vi "传感器数据.vi"() -> (0 "电机角度":sgl format="%#.3f", 1 "拉压力":sgl format="%#.3f", 2 "扭矩":sgl format="%#.3f", 3 "电缸位移":sgl format="%#.3f", 4 "电缸自带压力":sgl format="%#.3f", 5 "传感器读数":T1 {"Factorysensor2" format="%#.3f"; "输出轴移栽位移" format="%#.3f"; "输出轴旋转角度" format="%#.3f"; "Factorysensor" format="%#.3f"; "吸收电流" format="%#.3f"; "输出扭矩(大)" format="%#.3f"; "输出扭矩(小)" format="%#.3f"; "扭矩" format="%#.3f"; "输入编码位移" format="%#.3f"; "工装移载位移" format="%#.3f"; "输入移载位移" format="%#.3f"; "输入旋转位移" format="%#.3f"})   [LabVIEW 2020]
uses:
  Libraries/S7/S7.lvlib
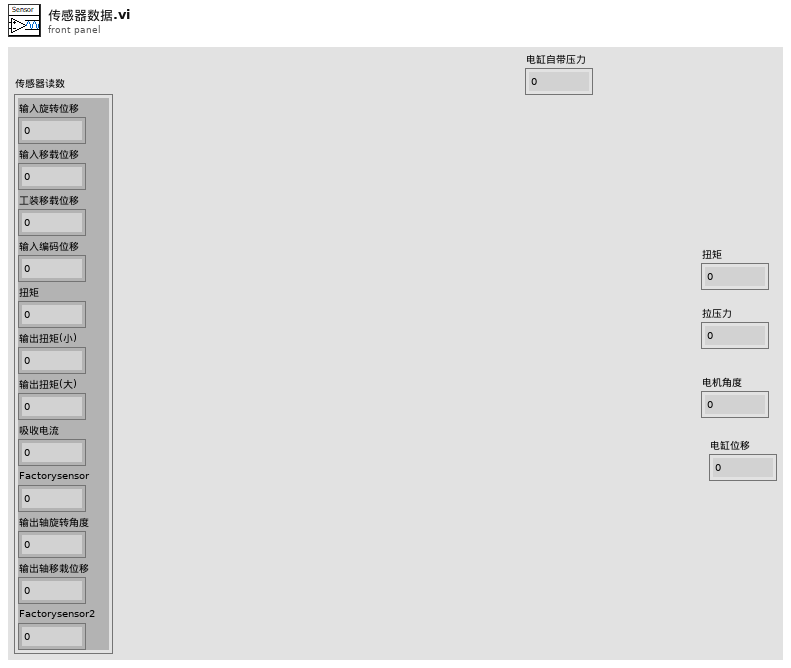
[diagram p1: front panel]
types:
  T1 = cluster{"输入旋转位移":sgl, "输入移载位移":sgl, "工装移载位移":sgl, "输入编码位移":sgl, "扭矩":sgl, "输出扭矩(小)":sgl, "输出扭矩(大)":sgl, "吸收电流":sgl, "Factorysensor":sgl, "输出轴旋转角度":sgl, "输出轴移栽位移":sgl, "Factorysensor2":sgl}
  T2 = cluster{"输入轴扭矩":dbl, "输出轴扭矩小量程":dbl, "输出轴扭矩大量程":dbl}
  T3 = typedef "S7.lvlib/Read_Data (Reply Payload)--cluster.ctl" = cluster{"读取成功":bool, "数据":u32[], "Read_Data_error":errorcluster}
  T4 = cluster{sgl, sgl, sgl, sgl, dbl, dbl, dbl, sgl, sgl, sgl, sgl, sgl}
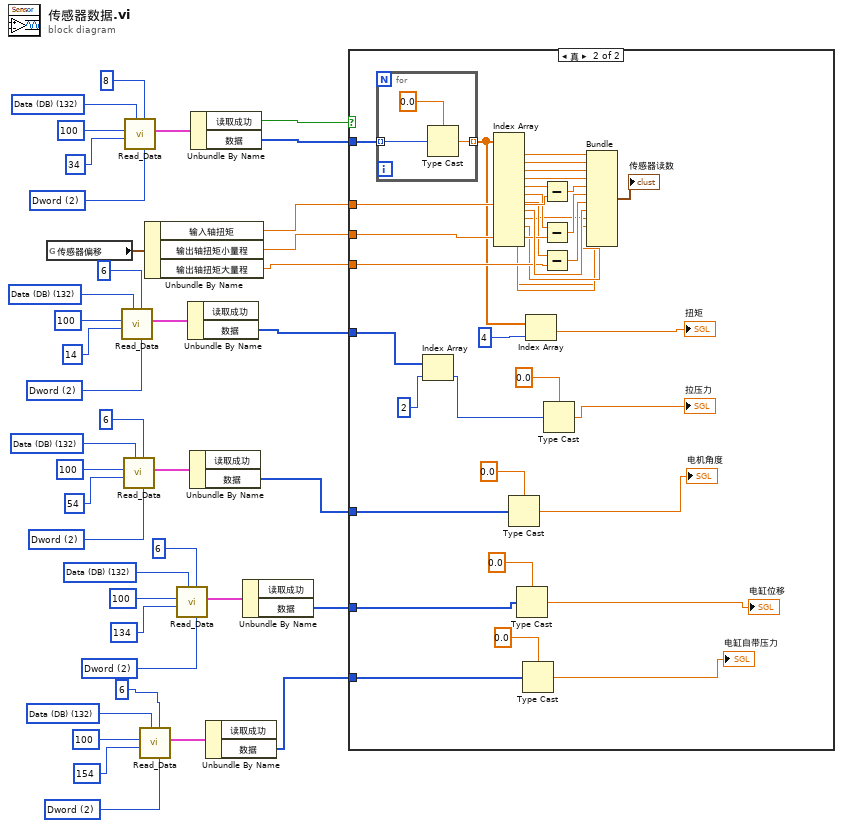
[diagram p0: block diagram]
diagram:
  w7 = u16 2 items=["byte", "word", "Dword"] ("数据类型")
  w5 = u8 132 items=["I/O (P)"=128, "Input (I)"=129, "Output (Q)"=130, "Bit Memory (M)"=131, "Data (DB)"=132, "Instance Data (DI)"=133, "Local Data (L)"=134, "Predecessor Local Data (VL)"=135] ("寄存器类型")
  w9 = u16 2 items=["byte", "word", "Dword"] ("数据类型")
  w12 = u8 132 items=["I/O (P)"=128, "Input (I)"=129, "Output (Q)"=130, "Bit Memory (M)"=131, "Data (DB)"=132, "Instance Data (DI)"=133, "Local Data (L)"=134, "Predecessor Local Data (VL)"=135] ("寄存器类型")
  w18 = u16 2 items=["byte", "word", "Dword"] ("数据类型")
  w19 = u8 132 items=["I/O (P)"=128, "Input (I)"=129, "Output (Q)"=130, "Bit Memory (M)"=131, "Data (DB)"=132, "Instance Data (DI)"=133, "Local Data (L)"=134, "Predecessor Local Data (VL)"=135] ("寄存器类型")
  w26 = u16 2 items=["byte", "word", "Dword"] ("数据类型")
  w25 = u8 132 items=["I/O (P)"=128, "Input (I)"=129, "Output (Q)"=130, "Bit Memory (M)"=131, "Data (DB)"=132, "Instance Data (DI)"=133, "Local Data (L)"=134, "Predecessor Local Data (VL)"=135] ("寄存器类型")
  w37 = u16 2 items=["byte", "word", "Dword"] ("数据类型")
  w38 = u8 132 items=["I/O (P)"=128, "Input (I)"=129, "Output (Q)"=130, "Bit Memory (M)"=131, "Data (DB)"=132, "Instance Data (DI)"=133, "Local Data (L)"=134, "Predecessor Local Data (VL)"=135] ("寄存器类型")
  n1 = global read "传感器偏移.vi" "传感器偏移"() -> (w32:T2)
  n2 = call "Read_Data.vi"("数据类型"=w26, "读取长度"=u16 6, "寄存器类型"=w25, "起始地址"=u32 14, "DB #"=u16 100) -> ("Reply Payload"=w28:T3)  [unwired: 4 in, 2 out]
  n3 = call "Read_Data.vi"("数据类型"=w18, "读取长度"=u16 6, "寄存器类型"=w19, "起始地址"=u32 54, "DB #"=u16 100) -> ("Reply Payload"=w16:T3)  [unwired: 4 in, 2 out]
  n4 = call "Read_Data.vi"("数据类型"=w37, "读取长度"=u16 8, "寄存器类型"=w38, "起始地址"=u32 34, "DB #"=u16 100) -> ("Reply Payload"=w35:T3)  [unwired: 4 in, 2 out]
  n5 = call "Read_Data.vi"("数据类型"=w7, "读取长度"=u16 6, "寄存器类型"=w5, "起始地址"=u32 154, "DB #"=u16 100) -> ("Reply Payload"=w3:T3)  [unwired: 4 in, 2 out]
  n6 = Unbundle By Name(w32) -> ("输入轴扭矩"=w31:dbl, "输出轴扭矩小量程"=w30:dbl, "输出轴扭矩大量程"=w29:dbl)
  n7 = call "Read_Data.vi"("数据类型"=w9, "读取长度"=u16 6, "寄存器类型"=w12, "起始地址"=u32 134, "DB #"=u16 100) -> ("Reply Payload"=w14:T3)  [unwired: 4 in, 2 out]
  n8 = Unbundle By Name(w28) -> ("数据"=w22:u32[])  [unwired: 1 out]
  n9 = Unbundle By Name(w16) -> ("数据"=w15:u32[])  [unwired: 1 out]
  n10 = Unbundle By Name(w35) -> ("读取成功"=w33:bool, "数据"=w34:u32[])
  n11 = Unbundle By Name(w3) -> ("数据"=w1:u32[])  [unwired: 1 out]
  n12 = Unbundle By Name(w14) -> ("数据"=w8:u32[])  [unwired: 1 out]
  n13 = case shown="真" w33 {
    tunnel: w34 -> [_ w77]
    tunnel: w31 -> [_ w68]
    tunnel: w30 -> [_ w67]
    tunnel: w29 -> [_ w63]
    tunnel: w22 -> [_ w54]
    tunnel: w15 -> [_ w48]
    tunnel: w8 -> [_ w45]
    tunnel: w1 -> [_ w42]
    frame False {
    }
    frame True {
      n14 = for {
        tunnel: w77 -> [w79] mode=indexing
        tunnel: [w78] -> w58 mode=indexing
        n15 = Type Cast(type=sgl 0.0, x=w79) -> (*(type *) &x=w78:sgl)
      }
      n16 = Index Array(array=w54, index=2 ("索引")) -> (element=w51:u32)
      n17 = Index Array(array=w58) -> (element #1=w76:sgl, element #2=w75:sgl, element #3=w74:sgl, element #4=w73:sgl, element #5=w72:sgl, element #6=w66:sgl, element #7=w64:sgl, element #8=w71:sgl, element #9=w61:sgl, element #10=w60:sgl, element #11=w59:sgl, element #12=w57:sgl)  [unwired: 12 in]
      n18 = Type Cast(type=sgl 0.0, x=w48) -> (*(type *) &x=→"电机角度":sgl)
      n19 = Type Cast(type=sgl 0.0, x=w45) -> (*(type *) &x=→"电缸位移":sgl)
      n20 = Type Cast(type=sgl 0.0, x=w42) -> (*(type *) &x=→"电缸自带压力":sgl)
      n21 = Index Array(array=w58, index=4 ("索引")) -> (element=→"扭矩":sgl)
      n22 = Subtract(x=w72, y=w68) -> (x-y=w69:dbl)
      n23 = Subtract(x=w66, y=w67) -> (x-y=w65:dbl)
      n24 = Subtract(x=w64, y=w63) -> (x-y=w62:dbl)
      n25 = Type Cast(type=sgl 0.0, x=w51) -> (*(type *) &x=→"拉压力":sgl)
      n26 = Bundle(w76, w75, w74, w73, w69, w65, w62, w71, w61, w60, w59, w57) -> (→"传感器读数":T4)  [unwired: 1 in]
    }
  }
